vi "shift register.vi"() -> ()   [LabVIEW 2015]
panel:
  out "loop 2":i32
  in  "loop":i32
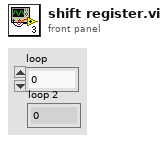
[diagram p1: front panel]
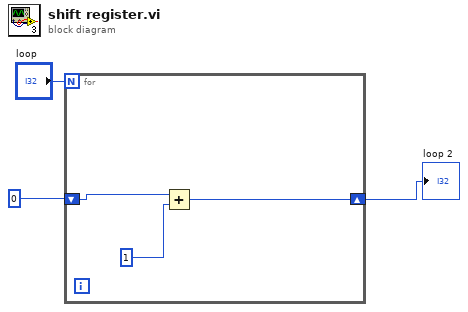
[diagram p0: block diagram]
diagram:
  n1 = for {
    N: "loop" -> [_]
    shift-right: [w4] -> w1
    shift-left: 0 -> [w6]
    n2 = Add(x=w6, y=1) -> (x+y=w4:i32)
  }
  "loop 2" <- w1
